vi "Read Key (Throw Error If Not Found) (String).vi"(8 "Error In":errorcluster, 9 "Key":string, 10 "Section":string, 11 "Config File Refnum in":T1) -> (0 "Error Out":errorcluster, 3 "Key Value":string)   [LabVIEW 2016, in "Error Manager.lvlib" / "Settings.lvclass"]
doc: "This VI reads the value of a config file (INI file) key. The VI throws an error with an informative error message if the key wasn't found."
uses:
  Settings.lvclass
  <vilib>/Utility/config.llb/NI_LVConfig.lvlib
  Error Manager.lvlib
  <vilib>/Utility/config.llb/Read Key (String).vi
  <vilib>/Utility/config.llb/Config Data RefNum.ctl
panel:
  # "Development\nControls or indicators that are useful for development or testing, but which are not outputs of the VI."
  # "Input\nInputs to the VI"
  # "Output\nOutputs of the VI"
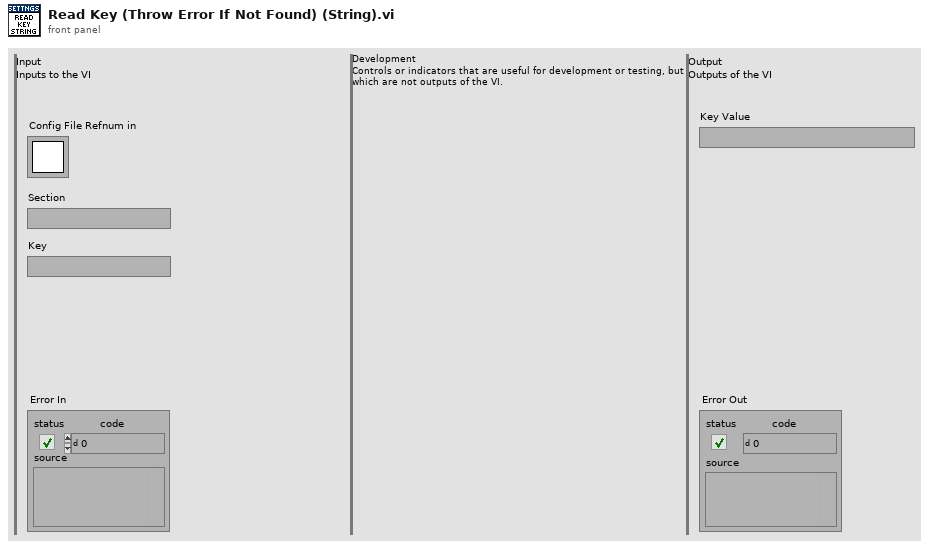
[diagram p1: front panel]
types:
  T1 = typedef "NI_LVConfig.lvlib/Config Data RefNum.ctl" = refnum<k1>
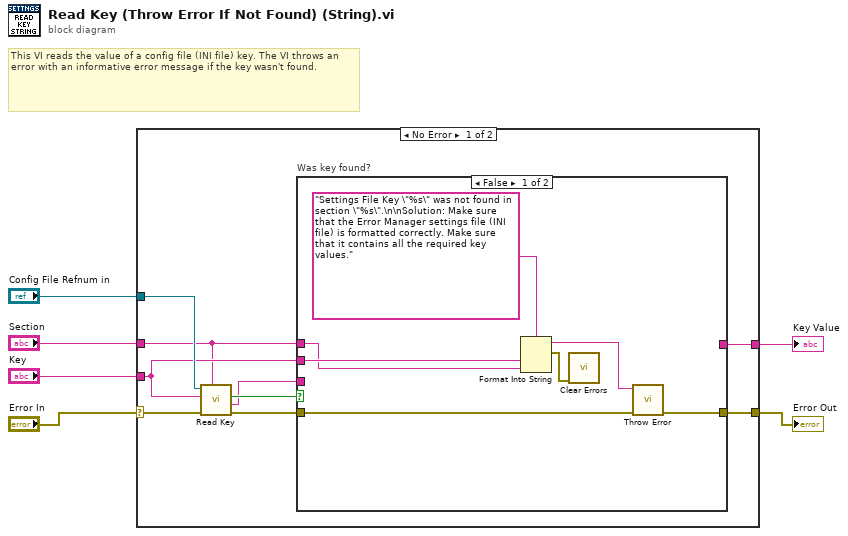
[diagram p0: block diagram]
diagram:
  # "This VI reads the value of a config file (INI file) key. The VI throws an error with an informative error message if the key wasn't found."
  n1 = case shown="No Error" "Error In" {
    selector: "Error In" -> [w13 w25]
    tunnel: [w12 w25] -> w5
    tunnel: "Config File Refnum in" -> [w11 _]
    tunnel: "Section" -> [w9 _]
    tunnel: "Key" -> [w10 _]
    tunnel: [w7 _] -> w1
    frame No Error {
      n2 = call-poly <vilib>:"Read Key.vi"("section"=w9, "error in (no error)"=w13, "key"=w10, "refnum"=w11) -> ("error out"=w15:errorcluster, "value"=w8:string, "found?"=w14:bool)  [unwired: 4 in, 1 out]
      n3 = case "Was key found?" shown="False" w14 {
        tunnel: w15 -> [w22 w24]
        tunnel: [w21 w24] -> w12
        tunnel: w10 -> [w17 _]
        tunnel: w9 -> [w16 _]
        tunnel: w8 -> [_ w23]
        tunnel: [_ w23] -> w7
        frame False {
          n4 = Format Into String(format string="Settings File Key \"%s\" was not found in section \"%s\".\n\nSolution: Make sure that the Error Manager settings file (INI file) is formatted correctly. Make sure that it contains all the required key values." ("section"), w17, w16) -> (resulting string=w19:string, error out=w18:errorcluster)  [unwired: 2 in]
          n5 = call <vilib>:"Clear Errors.vi"("error in (no error)"=w18) -> ()  [unwired: 5 in, 2 out]
          n6 = call "Throw Error.vi"("error in"=w22, "Error Message"=w19) -> ("error out"=w21:errorcluster)  [unwired: 9 in]
        }
        frame True {
        }
      }
    }
    frame Error {
    }
  }
  "Error Out" <- w5
  "Key Value" <- w1
